vi "Build Traverse Set.vi"(7 "Max Translation Output(0-1)":dbl=1.0, 11 "Traverse":T1 {"Angle" scale format="%.3f"; "Velocity" scale=-1.0..1.0 scale format="%.1f"}) -> (3 "Frame Rotation Set Out":T4 {"Back Right"."Angle" scale format="%.3f"; "Back Right"."Velocity" scale=-1.0..1.0 scale format="%.1f"; "Back Left"."Angle" scale format="%.3f"; "Back Left"."Velocity" scale=-1.0..1.0 scale format="%.1f"; "Front Left"."Angle" scale format="%.3f"; "Front Left"."Velocity" scale=-1.0..1.0 scale format="%.1f"; "Front Right"."Angle" scale format="%.3f"; "Front Right"."Velocity" scale=-1.0..1.0 scale format="%.1f"})   [LabVIEW 2023, in "SwerveDrive_ACT.lvlib"]
uses:
  SwerveDrive_ACT.lvlib
  Shared Code/TypeDefs/Cluster_Swerve 4 Steer and Velocity.ctl
  Shared Code/TypeDefs/Cluster_Module Velocity-Direction-Rotations.ctl
  Shared Code/TypeDefs/Level_Velocity plus-minus 1.ctl
  Shared Code/TypeDefs/Dial_Compase heading unit circle CCW positive.ctl
panel:
  # "\"Front\" of Robot"
  # "Right Hand Rule"
  # "X"
  # "+CCW"
  # "Y"
  # "(0,0)"
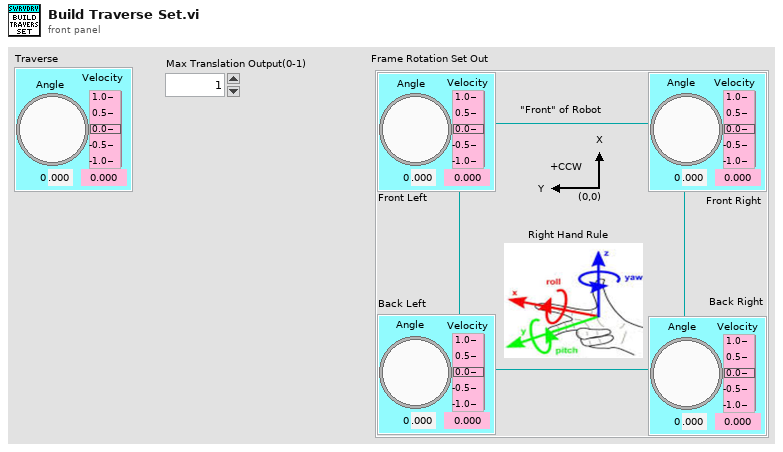
[diagram p1: front panel]
types:
  T1 = typedef "Cluster_Module Velocity-Direction-Rotations.ctl" = cluster{"Velocity":T2, "Angle":T3, "Rotations Count":dbl}
  T2 = typedef "Level_Velocity plus-minus 1.ctl" = dbl
  T3 = typedef "Dial_Compase heading unit circle CCW positive.ctl" = dbl
  T4 = typedef "Cluster_Swerve 4 Steer and Velocity.ctl" = cluster{"Front Right":T1, "Front Left":T1, "Back Left":T1, "Back Right":T1}
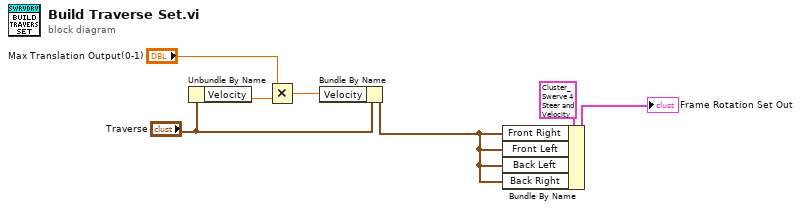
[diagram p0: block diagram]
diagram:
  n1 = Unbundle By Name("Traverse") -> ("Velocity"=w3:T2)
  n2 = Multiply(x="Max Translation Output(0-1)", y=w3) -> (x*y=w1:T2)
  n3 = Bundle By Name(cluster="Traverse", "Velocity"=w1) -> (w4:T1)
  n4 = Bundle By Name(cluster=T4 {"Front Right"={"Velocity"=0.0, "Angle"=0.0, "Rotations Count"=0.0}, "Front Left"={"Velocity"=0.0, "Angle"=0.0, "Rotations Count"=0.0}, "Back Left"={"Velocity"=0.0, "Angle"=0.0, "Rotations Count"=0.0}, "Back Right"={"Velocity"=0.0, "Angle"=0.0, "Rotations Count"=0.0}} ("Frame Rotation Set Out"), "Front Right"=w4, "Front Left"=w4, "Back Left"=w4, "Back Right"=w4) -> (→"Frame Rotation Set Out":T4)
